vi "Top_level.vi"() -> ()   [LabVIEW 2013]
uses:
  <vilib>/Utility/file.llb/Write To Spreadsheet File (DBL).vi
  <instrlib>/Tektronix FCA MCA 3000 Series/Tektronix FCA MCA 3000 Series.lvlib
panel:
  in  "Measure From":i32(ring) items=["A", "B", "C (HF-input option)", "E (Rear panel arming input)", "A prescaled by 2", "Internal Reference", "A with the variable hysteresis mode"]
  in  "Measure From":i32(ring) items=["A", "B", "C (HF-input option)", "E (Rear panel arming input)", "A prescaled by 2", "Internal Reference", "A with the variable hysteresis mode"]
  in  "Measure From":i32(ring) items=["A", "B", "C (HF-input option)", "E (Rear panel arming input)", "A prescaled by 2", "Internal Reference", "A with the variable hysteresis mode"]
  in  "File Name 3":string
  in  "Save Path 3":string
  out "Temperature Readings 3":cluster{"element":dbl, "element":dbl}[](graph)
  out "Frequency Readings 3":cluster{"X":dbl, "Y":dbl}[](graph)
  in  "arduino 3":refnum<visa-resource-name>
  in  "File Name 2":string
  in  "Save Path 2":string
  out "Temperature Readings 2":cluster{"element":dbl, "element":dbl}[](graph)
  out "Frequency Readings 2":cluster{"X":dbl, "Y":dbl}[](graph)
  in  "arduino 2":refnum<visa-resource-name>
  in  "File Name":string
  in  "Save Path":string
  out "Frequency Readings":cluster{"X":dbl, "Y":dbl}[](graph)
  in  "Number of Measurements (1)":i32=1
  in  "Frequency Generator":refnum<visa-resource-name>
  in  "stop":bool
  out "Temperature Readings":cluster{"element":dbl, "element":dbl}[](graph)
  in  "arduino 1":refnum<visa-resource-name>
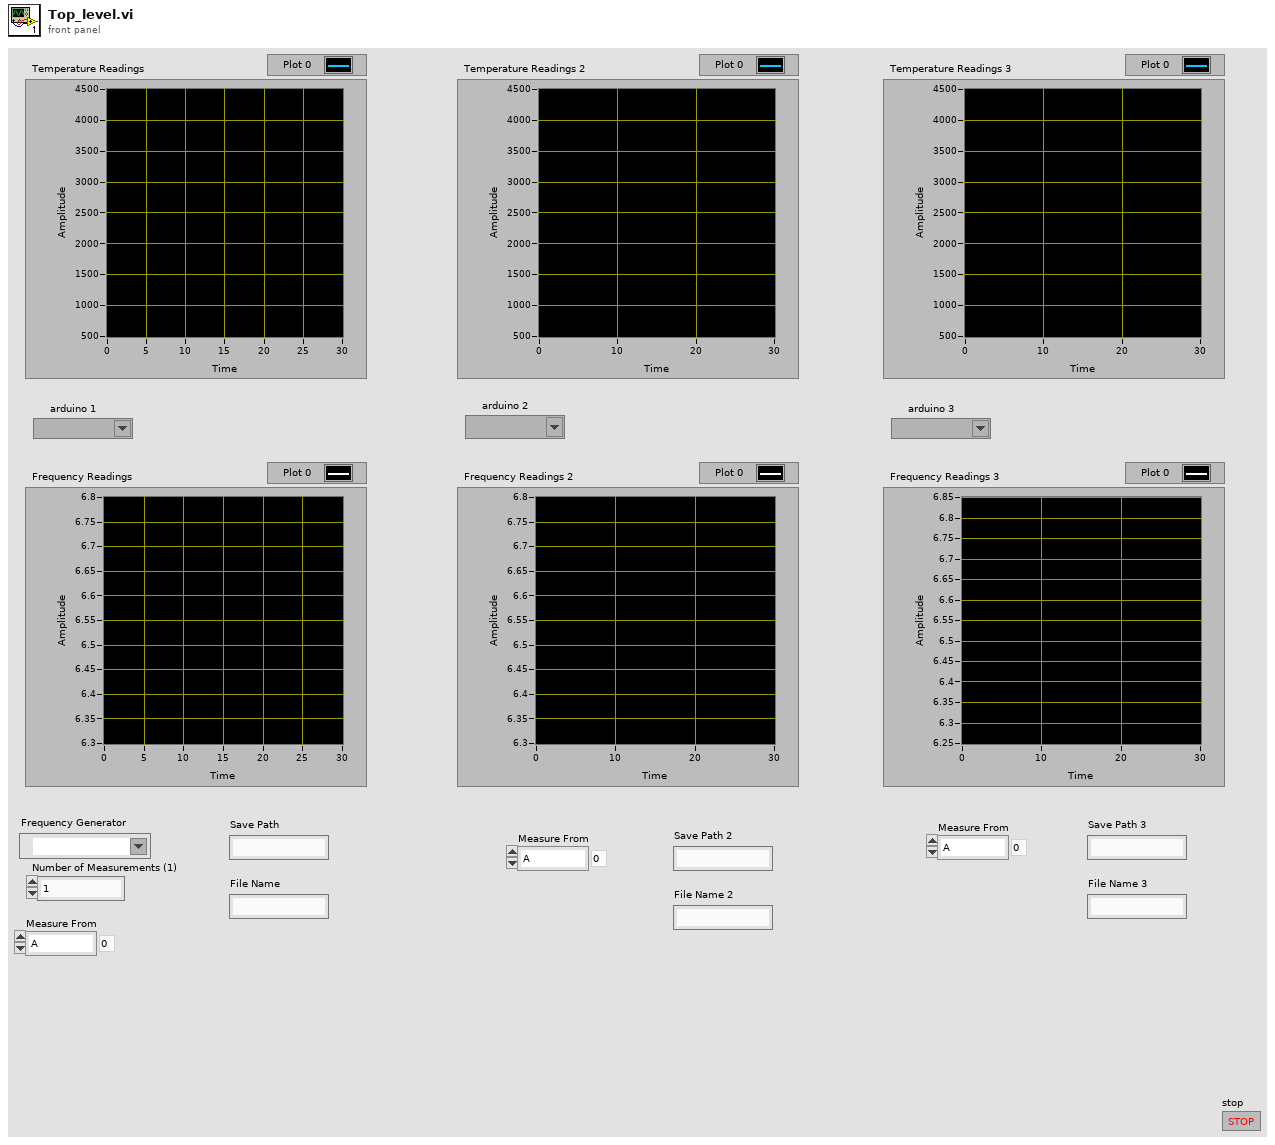
[diagram p1: front panel]
types:
  T1 = typedef "NI_Matrix.lvlib/RealMatrix.ctl" = dbl[][]
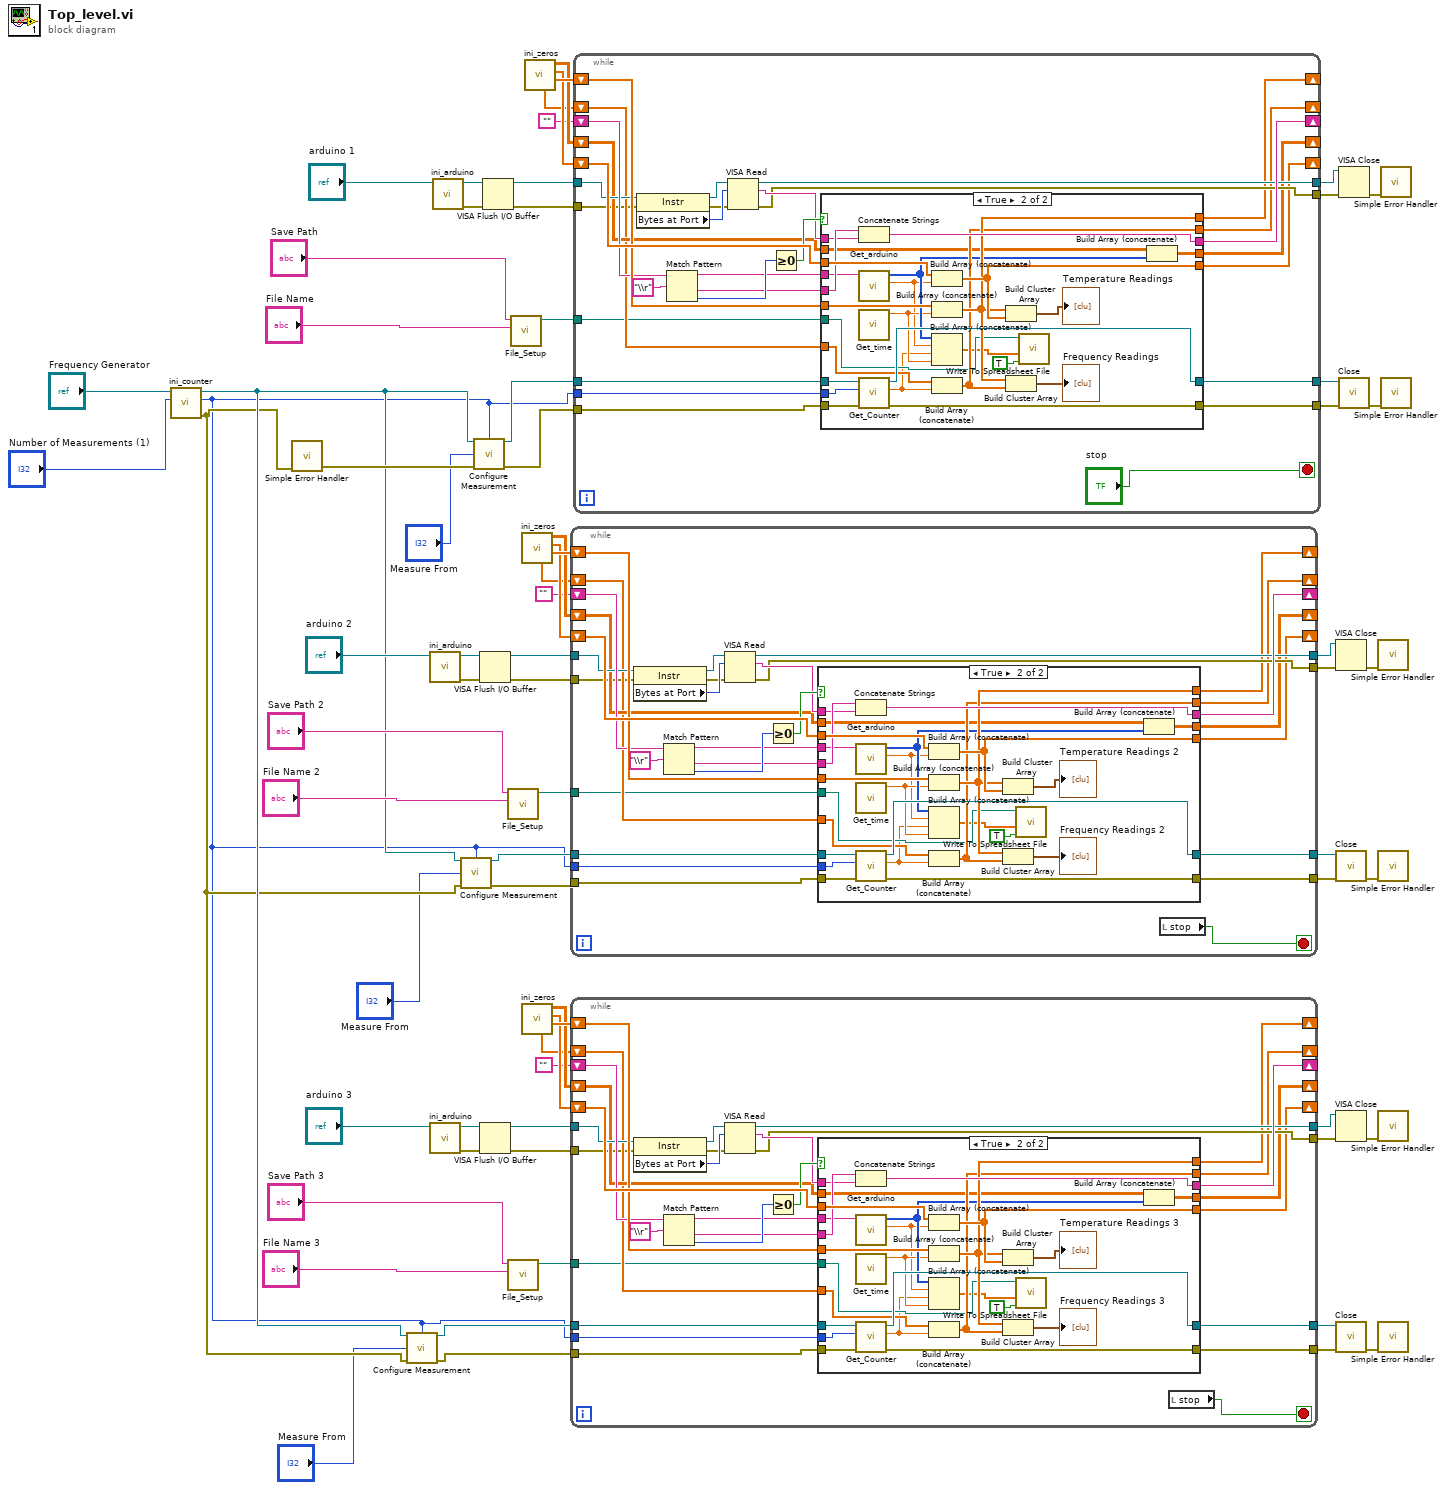
[diagram p0: block diagram]
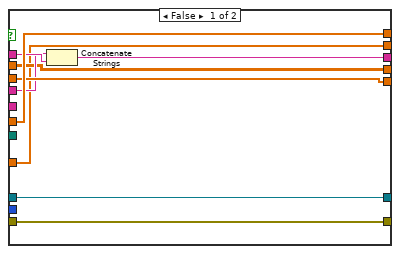
[diagram p2: hidden frame]
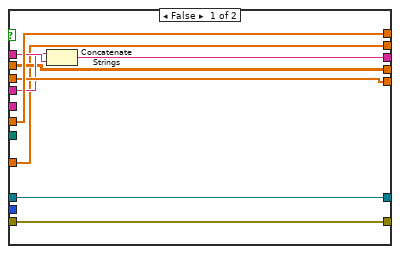
[diagram p3: hidden frame]
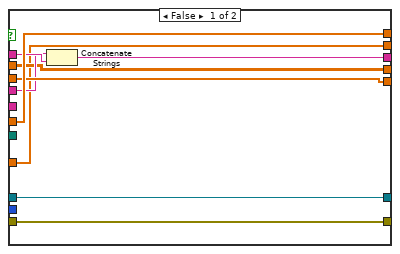
[diagram p4: hidden frame]
diagram:
  n1 = call "ini_counter.vi"("Number of Measurements (1) in"="Number of Measurements (1)", "VISA Refnum in"="Frequency Generator") -> ("error out"=w7:errorcluster, "Number of Measurements (1) out"=w4:i32, "VISA Refnum out"=w8:refnum<visa-resource-name>)  [unwired: 7 in]
  n2 = call <vilib>:"Simple Error Handler.vi"("error in (no error)"=w7) -> ("error out"=w11:errorcluster)  [unwired: 4 in, 4 out]
  n3 = call <instrlib>:"Configure Measurement.vi"("VISA resource name"=w8, "Number of Measurements (1)"=w4, "Channel  1 (0: A)"="Measure From", "error in (no error)"=w7) -> ("VISA resource name out"=w5:refnum<visa-resource-name>, "error out"=w6:errorcluster)  [unwired: 10 in]
  n4 = call "ini_arduino.vi"("VISA Refnum in"="arduino 2") -> ("error out"=w40:errorcluster, "VISA Refnum out"=w49:refnum<visa-resource-name>)  [unwired: 9 in]
  n5 = call "ini_arduino.vi"("VISA Refnum in"="arduino 3") -> ("error out"=w21:errorcluster, "VISA Refnum out"=w30:refnum<visa-resource-name>)  [unwired: 9 in]
  n6 = call "ini_arduino.vi"("VISA Refnum in"="arduino 1") -> ("error out"=w60:errorcluster, "VISA Refnum out"=w70:refnum<visa-resource-name>)  [unwired: 9 in]
  n7 = call <instrlib>:"Configure Measurement.vi"("VISA resource name"=w8, "Number of Measurements (1)"=w4, "Channel  1 (0: A)"="Measure From", "error in (no error)"=w7) -> ("VISA resource name out"=w10:refnum<visa-resource-name>, "error out"=w9:errorcluster)  [unwired: 10 in]
  n8 = call <instrlib>:"Configure Measurement.vi"("VISA resource name"=w8, "Number of Measurements (1)"=w4, "Channel  1 (0: A)"="Measure From", "error in (no error)"=w11) -> ("VISA resource name out"=w13:refnum<visa-resource-name>, "error out"=w12:errorcluster)  [unwired: 10 in]
  n9 = VISA Flush I/O Buffer(VISA resource name=w49, error in (no error)=w40) -> (VISA resource name out=w48:refnum<visa-resource-name>, error out=w39:errorcluster)  [unwired: 1 in]
  n10 = VISA Flush I/O Buffer(VISA resource name=w30, error in (no error)=w21) -> (VISA resource name out=w29:refnum<visa-resource-name>, error out=w20:errorcluster)  [unwired: 1 in]
  n11 = VISA Flush I/O Buffer(VISA resource name=w70, error in (no error)=w60) -> (VISA resource name out=w69:refnum<visa-resource-name>, error out=w59:errorcluster)  [unwired: 1 in]
  n12 = call "File_Setup.vi"("File Name"="File Name 2", "Save Path"="Save Path 2") -> ("new file path (Not A Path if cancelled)"=w33:path)  [unwired: 9 in]
  n13 = call "File_Setup.vi"("File Name"="File Name 3", "Save Path"="Save Path 3") -> ("new file path (Not A Path if cancelled)"=w14:path)  [unwired: 9 in]
  n14 = call "File_Setup.vi"("File Name"="File Name", "Save Path"="Save Path") -> ("new file path (Not A Path if cancelled)"=w53:path)  [unwired: 9 in]
  n15 = call "ini_zeros.vi"() -> ("Array 4"=w50:dbl[], "Array 3"=w47:dbl[], "Array 2"=w46:dbl[][], "Array"=w41:dbl[])  [unwired: 8 in]
  n16 = call "ini_zeros.vi"() -> ("Array 4"=w31:dbl[], "Array 3"=w28:dbl[], "Array 2"=w27:dbl[][], "Array"=w22:dbl[])  [unwired: 8 in]
  n17 = call "ini_zeros.vi"() -> ("Array 4"=w71:dbl[], "Array 3"=w68:dbl[], "Array 2"=w67:dbl[][], "Array"=w61:dbl[])  [unwired: 8 in]
  n18 = while {
    tunnel: w48 -> [w90]
    shift-right: [w77] -> _
    shift-left: w47 -> [w100]
    shift-right: [w75] -> _
    shift-left: w50 -> [w99]
    shift-right: [w91] -> _
    shift-left: "" -> [w98]
    shift-right: [w78] -> _
    shift-left: w46 -> [w89]
    tunnel: w10 -> [w88]
    tunnel: w9 -> [w87]
    tunnel: [w86] -> w43
    tunnel: [w85] -> w42
    tunnel: w4 -> [w84]
    shift-right: [w76] -> _
    shift-left: w41 -> [w83]
    tunnel: w39 -> [w82]
    tunnel: [w80] -> w38
    tunnel: [w79] -> w37
    tunnel: w33 -> [w74]
    stop <- w73 stop-if-true
    n19 = property class="Instr"(reference=w90, error in=w82) -> (reference out=w102:refnum<visa-resource-name>, error out=w81:errorcluster, "Bytes at Port"=w101:u32)
    n20 = Match Pattern(string=w98, regular expression="\\r") -> (before substring=w94:string, after substring=w93:string, offset past match=w95:i32)  [unwired: 1 in, 1 out]
    n21 = VISA Read(VISA resource name=w102, byte count=w101, error in (no error)=w81) -> (VISA resource name out=w80:refnum<visa-resource-name>, read buffer=w92:string, error out=w79:errorcluster)  [unwired: 1 out]
    n22 = Greater Or Equal To 0?(x=w95) -> (x >= 0?=w96:bool)
    n23 = case shown="True" w96 {
      tunnel: w94 -> [w108 w129]
      tunnel: w100 -> [w110 w137]
      tunnel: w99 -> [w111 w136]
      tunnel: [w110 w135] -> w77
      tunnel: [w111 w123] -> w75
      tunnel: w93 -> [_ w133]
      tunnel: w92 -> [w109 w132]
      tunnel: [w107 w131] -> w91
      tunnel: w89 -> [w106 w113]
      tunnel: [w106 w130] -> w78
      tunnel: w88 -> [w105 w112]
      tunnel: w87 -> [w104 w128]
      tunnel: [w105 w127] -> w86
      tunnel: [w104 w126] -> w85
      tunnel: w84 -> [_ w125]
      tunnel: w83 -> [w103 w124]
      tunnel: [w103 w122] -> w76
      tunnel: w74 -> [_ w119]
      frame False {
        n24 = Concatenate Strings(w108, w109) -> (w107:string)
      }
      frame True {
        n25 = Concatenate Strings(w133, w132) -> (w131:string)
        n26 = call "Get_arduino.vi"("String"=w129) -> ("mean"=w116:dbl, "Array"=w118:i32[])  [unwired: 9 in]
        n27 = call "Get_time.vi"() -> ("Elapsed Time (s)"=w117:dbl)  [unwired: 11 in]
        n28 = call "Get_Counter.vi"("error in (no error)"=w128, "Number of Measurements (1) in"=w125, "VISA Refnum in"=w112) -> ("error out"=w126:errorcluster, "Numeric"=w115:dbl, "VISA Refnum out"=w127:refnum<visa-resource-name>)  [unwired: 6 in]
        n29 = Build Array (concatenate)(w137, w116) -> (w135:dbl[])
        n30 = Build Array (concatenate)(w136, w117) -> (w123:dbl[])
        n31 = Build Array (concatenate)(w118, w116, w115, w117) -> (w114:dbl[])
        n32 = Build Array (concatenate)(w124, w115) -> (w122:dbl[])
        n33 = Build Cluster Array(w123, w135) -> (→"Temperature Readings 2":cluster{"Elapsed Time (s)":dbl, "mean":dbl}[])
        n34 = Build Cluster Array(w123, w122) -> (→"Frequency Readings 2":cluster{"Elapsed Time (s)":dbl, "Numeric":dbl}[])
        n35 = call-poly <vilib>:"Write To Spreadsheet File.vi"("append to file? (new file:F)"=TRUE, "1D data"=w114, "file path (dialog if empty)"=w119) -> ()  [unwired: 5 in, 1 out]
        n36 = Build Array (concatenate)(w113, w118) -> (w130:T1)
      }
    }
    n37 = local read "stop"() -> (w73:bool)
  }
  n38 = while {
    tunnel: w29 -> [w155]
    shift-right: [w142] -> _
    shift-left: w28 -> [w165]
    shift-right: [w140] -> _
    shift-left: w31 -> [w164]
    shift-right: [w156] -> _
    shift-left: "" -> [w163]
    shift-right: [w143] -> _
    shift-left: w27 -> [w154]
    tunnel: w5 -> [w153]
    tunnel: w6 -> [w152]
    tunnel: [w151] -> w24
    tunnel: [w150] -> w23
    tunnel: w4 -> [w149]
    shift-right: [w141] -> _
    shift-left: w22 -> [w148]
    tunnel: w20 -> [w147]
    tunnel: [w145] -> w19
    tunnel: [w144] -> w18
    tunnel: w14 -> [w139]
    stop <- w138 stop-if-true
    n39 = property class="Instr"(reference=w155, error in=w147) -> (reference out=w167:refnum<visa-resource-name>, error out=w146:errorcluster, "Bytes at Port"=w166:u32)
    n40 = Match Pattern(string=w163, regular expression="\\r") -> (before substring=w159:string, after substring=w158:string, offset past match=w160:i32)  [unwired: 1 in, 1 out]
    n41 = VISA Read(VISA resource name=w167, byte count=w166, error in (no error)=w146) -> (VISA resource name out=w145:refnum<visa-resource-name>, read buffer=w157:string, error out=w144:errorcluster)  [unwired: 1 out]
    n42 = Greater Or Equal To 0?(x=w160) -> (x >= 0?=w161:bool)
    n43 = case shown="True" w161 {
      tunnel: w159 -> [w173 w194]
      tunnel: w165 -> [w175 w202]
      tunnel: w164 -> [w176 w201]
      tunnel: [w175 w200] -> w142
      tunnel: [w176 w188] -> w140
      tunnel: w158 -> [_ w198]
      tunnel: w157 -> [w174 w197]
      tunnel: [w172 w196] -> w156
      tunnel: w154 -> [w171 w178]
      tunnel: [w171 w195] -> w143
      tunnel: w153 -> [w170 w177]
      tunnel: w152 -> [w169 w193]
      tunnel: [w170 w192] -> w151
      tunnel: [w169 w191] -> w150
      tunnel: w149 -> [_ w190]
      tunnel: w148 -> [w168 w189]
      tunnel: [w168 w187] -> w141
      tunnel: w139 -> [_ w184]
      frame False {
        n44 = Concatenate Strings(w173, w174) -> (w172:string)
      }
      frame True {
        n45 = Concatenate Strings(w198, w197) -> (w196:string)
        n46 = call "Get_arduino.vi"("String"=w194) -> ("mean"=w181:dbl, "Array"=w183:i32[])  [unwired: 9 in]
        n47 = call "Get_time.vi"() -> ("Elapsed Time (s)"=w182:dbl)  [unwired: 11 in]
        n48 = call "Get_Counter.vi"("error in (no error)"=w193, "Number of Measurements (1) in"=w190, "VISA Refnum in"=w177) -> ("error out"=w191:errorcluster, "Numeric"=w180:dbl, "VISA Refnum out"=w192:refnum<visa-resource-name>)  [unwired: 6 in]
        n49 = Build Array (concatenate)(w202, w181) -> (w200:dbl[])
        n50 = Build Array (concatenate)(w201, w182) -> (w188:dbl[])
        n51 = Build Array (concatenate)(w183, w181, w180, w182) -> (w179:dbl[])
        n52 = Build Array (concatenate)(w189, w180) -> (w187:dbl[])
        n53 = Build Cluster Array(w188, w200) -> (→"Temperature Readings 3":cluster{"Elapsed Time (s)":dbl, "mean":dbl}[])
        n54 = Build Cluster Array(w188, w187) -> (→"Frequency Readings 3":cluster{"Elapsed Time (s)":dbl, "Numeric":dbl}[])
        n55 = call-poly <vilib>:"Write To Spreadsheet File.vi"("append to file? (new file:F)"=TRUE, "1D data"=w179, "file path (dialog if empty)"=w184) -> ()  [unwired: 5 in, 1 out]
        n56 = Build Array (concatenate)(w178, w183) -> (w195:T1)
      }
    }
    n57 = local read "stop"() -> (w138:bool)
  }
  n58 = while {
    tunnel: w69 -> [w220]
    shift-right: [w207] -> _
    shift-left: w68 -> [w230]
    shift-right: [w205] -> _
    shift-left: w71 -> [w229]
    shift-right: [w221] -> _
    shift-left: "" -> [w228]
    shift-right: [w208] -> _
    shift-left: w67 -> [w219]
    tunnel: w13 -> [w218]
    tunnel: w12 -> [w217]
    tunnel: [w216] -> w63
    tunnel: [w215] -> w62
    tunnel: w4 -> [w214]
    shift-right: [w206] -> _
    shift-left: w61 -> [w213]
    tunnel: w59 -> [w212]
    tunnel: [w210] -> w58
    tunnel: [w209] -> w57
    tunnel: w53 -> [w204]
    stop <- "stop" stop-if-true
    n59 = property class="Instr"(reference=w220, error in=w212) -> (reference out=w232:refnum<visa-resource-name>, error out=w211:errorcluster, "Bytes at Port"=w231:u32)
    n60 = Match Pattern(string=w228, regular expression="\\r") -> (before substring=w224:string, after substring=w223:string, offset past match=w225:i32)  [unwired: 1 in, 1 out]
    n61 = VISA Read(VISA resource name=w232, byte count=w231, error in (no error)=w211) -> (VISA resource name out=w210:refnum<visa-resource-name>, read buffer=w222:string, error out=w209:errorcluster)  [unwired: 1 out]
    n62 = Greater Or Equal To 0?(x=w225) -> (x >= 0?=w226:bool)
    n63 = case shown="True" w226 {
      tunnel: w224 -> [w238 w259]
      tunnel: w230 -> [w240 w267]
      tunnel: w229 -> [w241 w266]
      tunnel: [w240 w265] -> w207
      tunnel: [w241 w253] -> w205
      tunnel: w223 -> [_ w263]
      tunnel: w222 -> [w239 w262]
      tunnel: [w237 w261] -> w221
      tunnel: w219 -> [w236 w243]
      tunnel: [w236 w260] -> w208
      tunnel: w218 -> [w235 w242]
      tunnel: w217 -> [w234 w258]
      tunnel: [w235 w257] -> w216
      tunnel: [w234 w256] -> w215
      tunnel: w214 -> [_ w255]
      tunnel: w213 -> [w233 w254]
      tunnel: [w233 w252] -> w206
      tunnel: w204 -> [_ w249]
      frame False {
        n64 = Concatenate Strings(w238, w239) -> (w237:string)
      }
      frame True {
        n65 = Concatenate Strings(w263, w262) -> (w261:string)
        n66 = call "Get_arduino.vi"("String"=w259) -> ("mean"=w246:dbl, "Array"=w248:i32[])  [unwired: 9 in]
        n67 = call "Get_time.vi"() -> ("Elapsed Time (s)"=w247:dbl)  [unwired: 11 in]
        n68 = call "Get_Counter.vi"("error in (no error)"=w258, "Number of Measurements (1) in"=w255, "VISA Refnum in"=w242) -> ("error out"=w256:errorcluster, "Numeric"=w245:dbl, "VISA Refnum out"=w257:refnum<visa-resource-name>)  [unwired: 6 in]
        n69 = Build Array (concatenate)(w267, w246) -> (w265:dbl[])
        n70 = Build Array (concatenate)(w266, w247) -> (w253:dbl[])
        n71 = Build Array (concatenate)(w248, w246, w245, w247) -> (w244:dbl[])
        n72 = Build Array (concatenate)(w254, w245) -> (w252:dbl[])
        n73 = Build Cluster Array(w253, w265) -> (→"Temperature Readings":cluster{"Elapsed Time (s)":dbl, "mean":dbl}[])
        n74 = Build Cluster Array(w253, w252) -> (→"Frequency Readings":cluster{"Elapsed Time (s)":dbl, "Numeric":dbl}[])
        n75 = call-poly <vilib>:"Write To Spreadsheet File.vi"("append to file? (new file:F)"=TRUE, "1D data"=w244, "file path (dialog if empty)"=w249) -> ()  [unwired: 5 in, 1 out]
        n76 = Build Array (concatenate)(w243, w248) -> (w260:T1)
      }
    }
  }
  n77 = VISA Close(VISA resource name=w38, error in (no error)=w37) -> (error out=w36:errorcluster)
  n78 = call <instrlib>:"Close.vi"("error in (no error)"=w42, "VISA resource name"=w43) -> ("error out"=w44:errorcluster)  [unwired: 9 in]
  n79 = VISA Close(VISA resource name=w19, error in (no error)=w18) -> (error out=w17:errorcluster)
  n80 = call <instrlib>:"Close.vi"("error in (no error)"=w23, "VISA resource name"=w24) -> ("error out"=w25:errorcluster)  [unwired: 9 in]
  n81 = VISA Close(VISA resource name=w58, error in (no error)=w57) -> (error out=w56:errorcluster)
  n82 = call <instrlib>:"Close.vi"("error in (no error)"=w62, "VISA resource name"=w63) -> ("error out"=w64:errorcluster)  [unwired: 9 in]
  n83 = call <vilib>:"Simple Error Handler.vi"("error in (no error)"=w36) -> ()  [unwired: 4 in, 5 out]
  n84 = call <vilib>:"Simple Error Handler.vi"("error in (no error)"=w44) -> ()  [unwired: 4 in, 5 out]
  n85 = call <vilib>:"Simple Error Handler.vi"("error in (no error)"=w17) -> ()  [unwired: 4 in, 5 out]
  n86 = call <vilib>:"Simple Error Handler.vi"("error in (no error)"=w25) -> ()  [unwired: 4 in, 5 out]
  n87 = call <vilib>:"Simple Error Handler.vi"("error in (no error)"=w56) -> ()  [unwired: 4 in, 5 out]
  n88 = call <vilib>:"Simple Error Handler.vi"("error in (no error)"=w64) -> ()  [unwired: 4 in, 5 out]
